vi "Value to U16 string.vi"(1 "Value":u16) -> (0 "U16 str (Little Endian)":string)   [LabVIEW 2015]
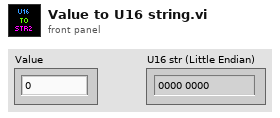
[diagram p1: front panel]
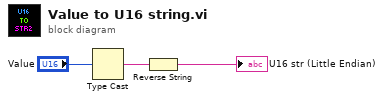
[diagram p0: block diagram]
diagram:
  n1 = Type Cast(x="Value") -> (*(type *) &x=w2:string)  [unwired: 1 in]
  n2 = Reverse String(1:w2) -> (0:→"U16 str (Little Endian)":string)
